vi "Basic Test 2.vi"() -> ()   [LabVIEW 2014, in "ESP8266 WiFi Wrapper.lvlib"]
uses:
  <vilib>/Aledyne-TSXperts/Arduino Compatible Compiler for LabVIEW/addons/ESP8266 WiFi Wrapper/ESP8266 WiFi Wrapper.lvlib
  <vilib>/Aledyne-TSXperts/Arduino Compatible Compiler for LabVIEW/Arduino Compatible Compiler for LabVIEW.lvlib
panel:
  in  "Listen Port":u8=80
  in  "WiFi Server Mode":T1(ring)=enum."WIFI_AP"
  in  "Password":string="secretcave"
  in  "SSID":string="SecretCave with Apples"
  out "Error Out":errorcluster
  in  "Error In":errorcluster
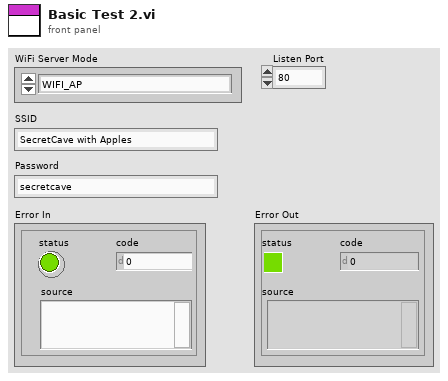
[diagram p1: front panel]
types:
  T1 = enum16{"WIFI_OFF", "WIFI_STA", "WIFI_AP", "WIFI_AP_STA"}
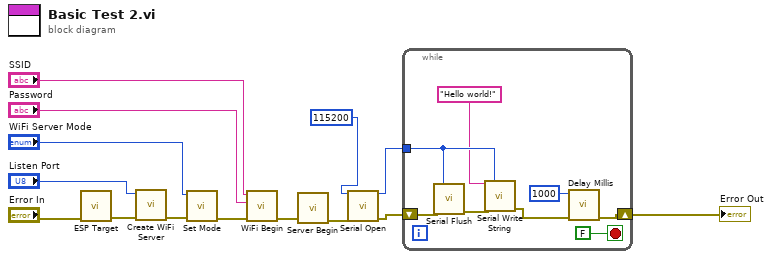
[diagram p0: block diagram]
diagram:
  n1 = call <vilib>:"ESP Target.vi"("Error In"="Error In") -> ("Error Out"=w2:errorcluster)  [unwired: 10 in]
  n2 = call <vilib>:"Create WiFi Server.vi"("Error In"=w2, "Listen Port"="Listen Port") -> ("Error Out"=w14:errorcluster)  [unwired: 9 in]
  n3 = call <vilib>:"Set Mode.vi"("Error In"=w14, "WiFi Server Mode"="WiFi Server Mode") -> ("Error Out"=w13:errorcluster)  [unwired: 9 in]
  n4 = call <vilib>:"WiFi Begin.vi"("Error In"=w13, "Password"="Password", "SSID"="SSID") -> ("Error Out"=w8:errorcluster)  [unwired: 8 in]
  n5 = call <vilib>:"Server Begin.vi"("Error In"=w8) -> ("Error Out"=w6:errorcluster)  [unwired: 10 in]
  n6 = call <vilib>:"Serial Open.vi"("Speed"=u32 115200, "error in (no error)"=w6) -> ("Instance"=w3:u8, "error out"=w5:errorcluster)  [unwired: 12 in]
  n7 = while {
    shift-right: [w22] -> w7
    shift-left: w5 -> [w19]
    tunnel: w3 -> [w16]
    stop <- FALSE stop-if-true
    n8 = call <vilib>:"Serial Flush.vi"("Instance"=w16, "error in (no error)"=w19) -> ("error out"=w18:errorcluster)  [unwired: 13 in]
    n9 = call <vilib>:"Serial Write String.vi"("String"="Hello world!", "Instance"=w16, "error in (no error)"=w18) -> ("error out"=w17:errorcluster)  [unwired: 12 in]
    n10 = call <vilib>:"Delay Millis.vi"("error in (no error)"=w17, "delay"=u32 1000) -> ("error out"=w22:errorcluster)  [unwired: 9 in]
  }
  "Error Out" <- w7
